vi "Double_GeneralGearShift_WithDeadTime.vi"(6 "error In":errorcluster, 7 "ShifterRef":T1={"DevStatus"={"status"=FALSE, "code"=0, "source"=""}, "Pneumatics Control Module"=0, "Forward Solenoid Channel"=enum."Invalid", "Reverse Solenoid Channel"=enum."Invalid"}, 9 "Shift Value":T3, 10 "Right":dbl, 11 "Left":dbl) -> (0 "error out":errorcluster, 1 "Shifting":bool, 2 "Right Output":dbl, 3 "Left Output":dbl)   [LabVIEW 2017]
uses:
  <vilib>/Rock Robotics/WPI/Solenoid/WPI_SolenoidValue.ctl
  <vilib>/Rock Robotics/WPI/Solenoid/WPI_SolenoidDevRef.ctl
  <vilib>/Rock Robotics/WPI/Solenoid/WPI_SolenoidChannel.ctl
  <vilib>/Rock Robotics/WPI/ThirdParty/Phoenix-LabVIEW/Motor Controller/Controls/CTRE_Phoenix_MotorControl_NeutralMode.ctl
  <vilib>/Rock Robotics/WPI/Solenoid/WPI_SolenoidSetEnum.vi
panel:
  out "Right Starting Point":dbl
  out "Left Starting Point":dbl
  out "TempTimeVal":u32
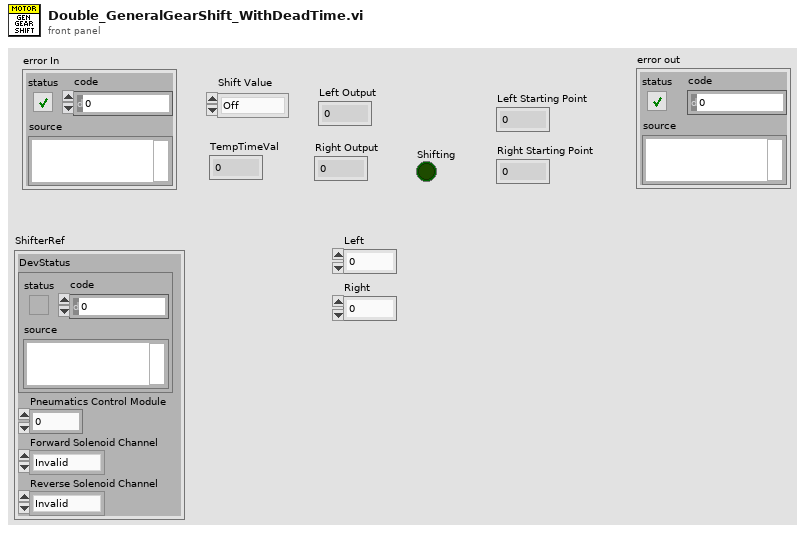
[diagram p1: front panel]
types:
  T1 = typedef "WPI_SolenoidDevRef.ctl" = cluster{"DevStatus":errorcluster, "Pneumatics Control Module":u8, "Forward Solenoid Channel":T2, "Reverse Solenoid Channel":T2}
  T2 = typedef "WPI_SolenoidChannel.ctl" = enum8{"Solenoid 0", "Solenoid 1", "Solenoid 2", "Solenoid 3", "Solenoid 4", "Solenoid 5", "Solenoid 6", "Solenoid 7", "Invalid"}
  T3 = typedef "WPI_SolenoidValue.ctl" = enum16{"Off", "On", "Forward", "Reverse"}
  T4 = typedef "WPI_MotorControlDeviceRef.ctl" = cluster{"DeviceStatus":errorcluster, "Type":T5, "PWM":cluster{"PWM Channel":T6, "DeadBand":T7}, "CAN":cluster{"Device Number":u8, "SetOutput VI Ref":variant, "GetOutput VI Ref":variant, "Enable VI Ref":variant, "Disable VI Ref":variant, "Data":variant}, "Invert":bool, "DIO PWM":cluster{"PWM \"Enable\" Channel":T6, "DIOChannel":T8, "PWM Rate":dbl}}
  T5 = typedef "WPI_MotorControlType.ctl" = enum16{"PWM", "CAN", "DIO PWM"}
  T6 = typedef "FPGA_DIOPWMChannel.ctl" = enum8{"PWM 0", "PWM 1", "PWM 2", "PWM 3", "PWM 4", "PWM 5", "PWM 6", "PWM 7", "PWM 8", "PWM 9", "PWM MXP 0", "PWM MXP 1", "PWM MXP 2", "PWM MXP 3", "PWM MXP 4", "PWM MXP 5", "PWM MXP 6", "PWM MXP 7", "PWM MXP 8", "PWM MXP 9", "Invalid"}
  T7 = typedef "WPI_PWMDeadband.ctl" = cluster{"Name":string, "maxPositivePwm":i32, "minPositivePwm":i32, "centerPwm":i32, "maxNegativePwm":i32, "minNegativePwm":i32, "angularRange":u16}
  T8 = typedef "FPGA_DIOChannel.ctl" = enum8{"DIO 0", "DIO 1", "DIO 2", "DIO 3", "DIO 4", "DIO 5", "DIO 6", "DIO 7", "DIO 8", "DIO 9", "DIO MXP 0", "DIO MXP 1", "DIO MXP 2", "DIO MXP 3", "DIO MXP 4", "DIO MXP 5", "DIO MXP 6", "DIO MXP 7", "DIO MXP 8", "DIO MXP 9", "DIO MXP 10", "DIO MXP 11", "DIO MXP 12", "DIO MXP 13", "DIO MXP 14", "DIO MXP 15", "SPI Port CS1", "SPI Port CS2", "SPI Port CS3", "SPI Port MISO", "SPI Port MOSI", "Invalid"}
  T9 = typedef "CTRE_Phoenix_MotorControl_NeutralMode.ctl" = enum8{"EEPROMSetting", "Override to Coast", "Override to Brake"}
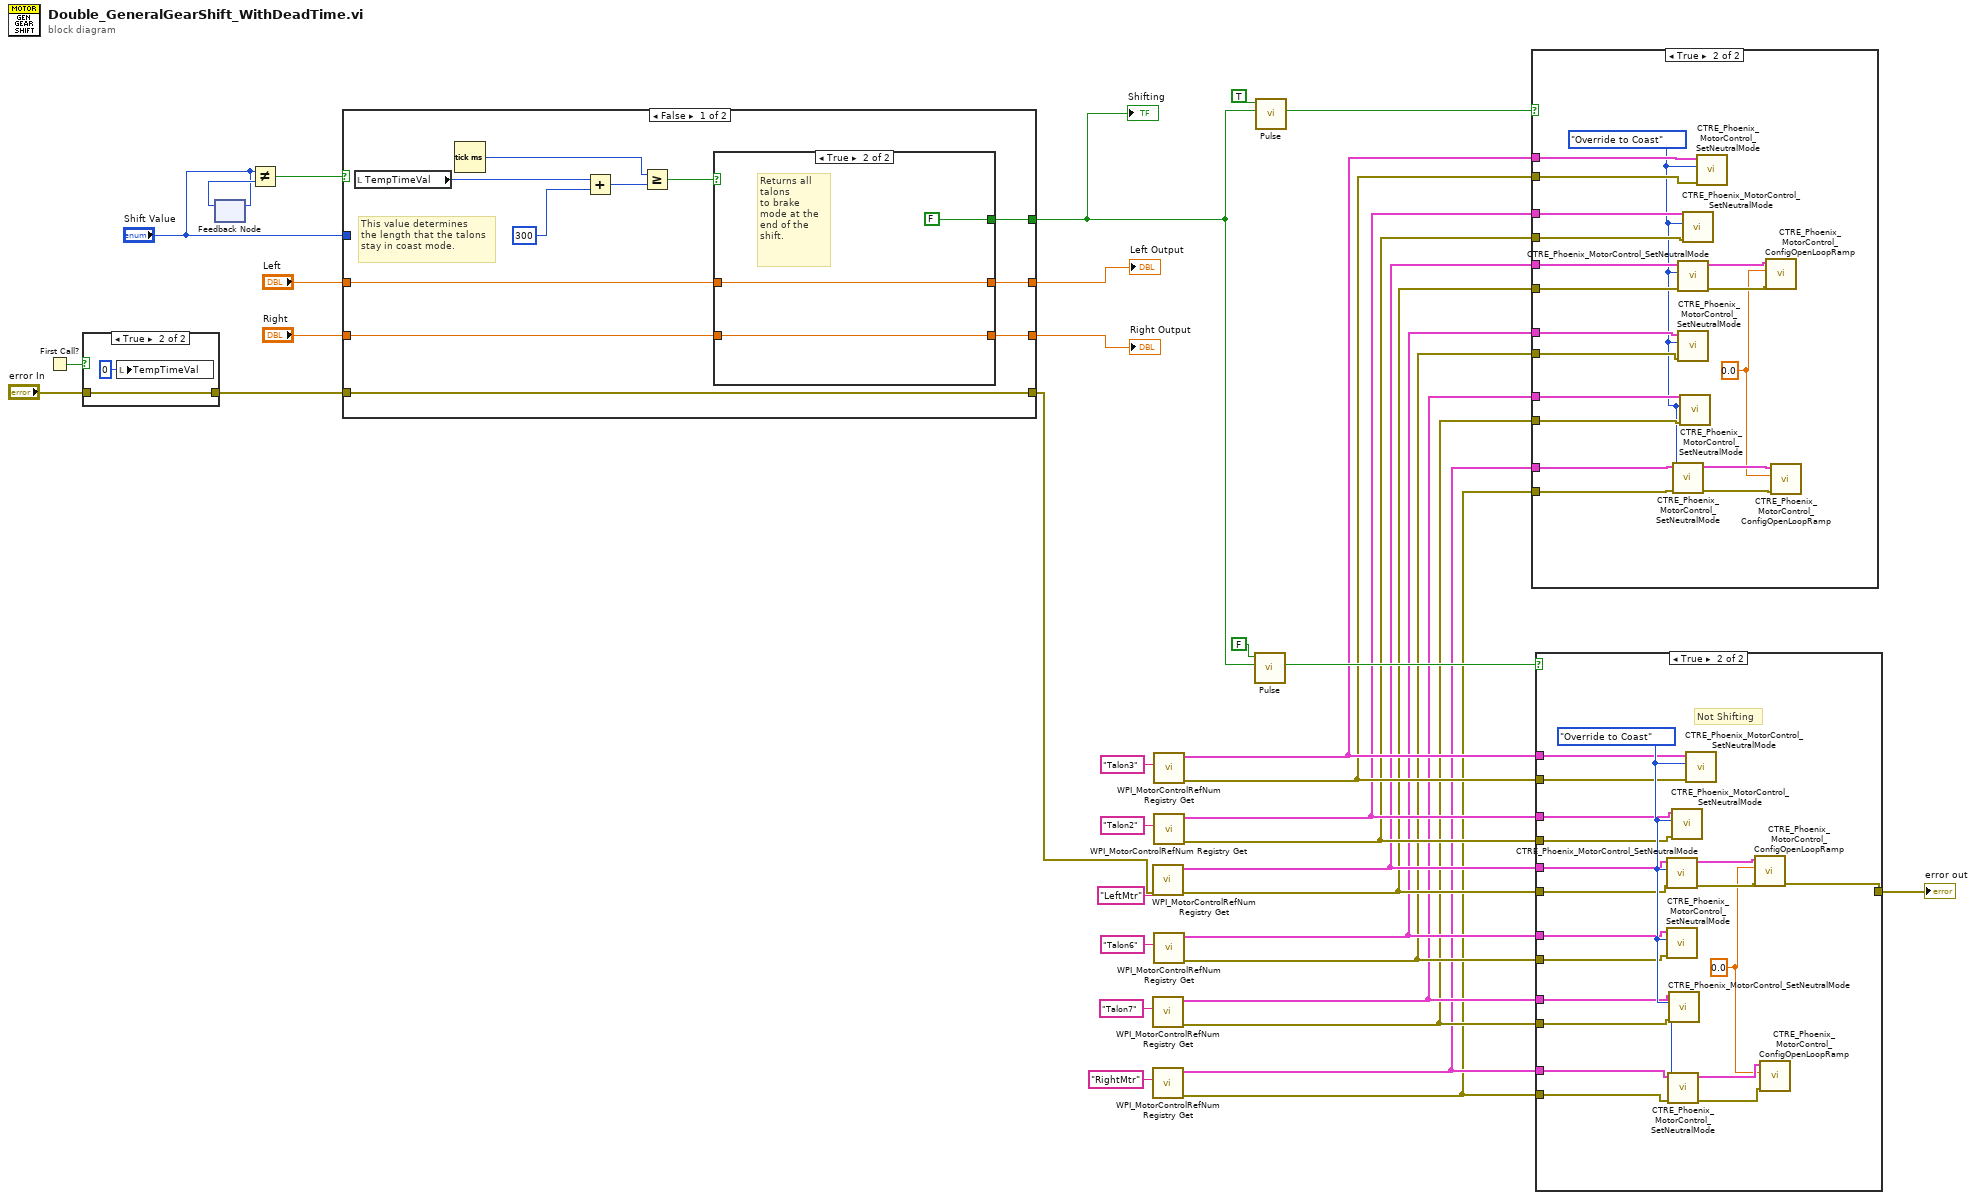
[diagram p0: block diagram]
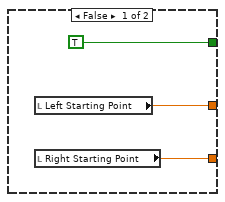
[diagram p5: hidden frame]
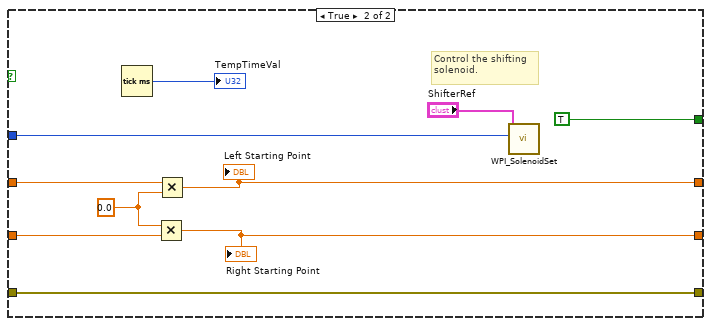
[diagram p6: hidden frame]
diagram:
  n1 = First Call?() -> (First Call?: T/F=w31:bool)
  n2 = case shown="True" w31 {
    tunnel: [w36 w37] -> w3
    tunnel: "error In" -> [w36 w37]
    frame False {
    }
    frame True {
      n3 = local write "TempTimeVal"(u32 0 ("TempTimeVal")) -> ()
    }
  }
  n4 = feedback-in #1("Shift Value") -> ()
  n5 = feedback #1() -> (w29:T3)  [unwired: 1 in]
  n6 = Not Equal?(x="Shift Value", y=w29) -> (x != y?=w28:bool)
  n7 = case shown="False" w28 {
    tunnel: [w49 w61] -> w35
    tunnel: [w48 w60] -> w34
    tunnel: "Right" -> [w47 w63]
    tunnel: "Left" -> [w46 w64]
    tunnel: [w40 TRUE] -> w23
    tunnel: "Shift Value" -> [_ w57]
    tunnel: w3 -> [w39 w56]
    tunnel: [w39 w56] -> w1
    frame False {
      # "This value determines\nthe length that the talons\nstay in coast mode."
      n8 = local read "TempTimeVal"() -> (w42:u32)
      n9 = Tick Count (ms)() -> (millisecond timer value=w44:u32)
      n10 = Add(x=w42, y=300) -> (x+y=w43:u32)
      n11 = Greater Or Equal?(x=w44, y=w43) -> (x >= y?=w45:bool)
      n12 = case shown="True" w45 {
        tunnel: [w51 w54] -> w49
        tunnel: [w52 w55] -> w48
        tunnel: w47 -> [_ w55]
        tunnel: w46 -> [_ w54]
        tunnel: [TRUE FALSE] -> w40
        frame False {
          n13 = local read "Left Starting Point"() -> (w51:dbl)
          n14 = local read "Right Starting Point"() -> (w52:dbl)
        }
        frame True {
          # "Returns all talons\nto brake mode at the\nend of the shift."
        }
      }
    }
    frame True {
      w62 = 0.0
      # "Control the shifting\nsolenoid."
      n15 = Tick Count (ms)() -> (millisecond timer value=→"TempTimeVal":u32)
      n16 = Multiply(x=w62, y=w63) -> (x*y=w60:dbl)
      "Right Starting Point" <- w60
      n17 = Multiply(x=w64, y=w62) -> (x*y=w61:dbl)
      "Left Starting Point" <- w61
      n18 = call-poly <vilib>:"WPI_SolenoidSet.vi"("Value"=w57, "SolenoidDevRef"="ShifterRef") -> ()  [unwired: 8 in, 2 out]
    }
  }
  "Left Output" <- w35
  "Right Output" <- w34
  "Shifting" <- w23
  n19 = call <vilib>:"WPI_MotorControlRefNum Registry Get.vi"("error in (no error)"=w1, "refnum name"="LeftMtr") -> ("error out"=w11:errorcluster, "MotorControlDevRef"=w12:T4)  [unwired: 8 in]
  n20 = call <vilib>:"WPI_MotorControlRefNum Registry Get.vi"("refnum name"="Talon7") -> ("error out"=w7:errorcluster, "MotorControlDevRef"=w8:T4)  [unwired: 9 in]
  n21 = call <vilib>:"WPI_MotorControlRefNum Registry Get.vi"("refnum name"="RightMtr") -> ("error out"=w5:errorcluster, "MotorControlDevRef"=w6:T4)  [unwired: 9 in]
  n22 = call <vilib>:"WPI_MotorControlRefNum Registry Get.vi"("refnum name"="Talon3") -> ("error out"=w15:errorcluster, "MotorControlDevRef"=w16:T4)  [unwired: 9 in]
  n23 = call <vilib>:"WPI_MotorControlRefNum Registry Get.vi"("refnum name"="Talon2") -> ("error out"=w13:errorcluster, "MotorControlDevRef"=w14:T4)  [unwired: 9 in]
  n24 = call <vilib>:"WPI_MotorControlRefNum Registry Get.vi"("refnum name"="Talon6") -> ("error out"=w9:errorcluster, "MotorControlDevRef"=w10:T4)  [unwired: 9 in]
  n25 = call "Pulse.vi"("Input"=w23, "Rising Edge?"=FALSE) -> ("Output"=w25:bool)  [unwired: 9 in]
  n26 = call "Pulse.vi"("Input"=w23, "Rising Edge?"=TRUE) -> ("Output"=w4:bool)  [unwired: 9 in]
  n27 = case shown="True" w4 {
    tunnel: w16 -> [_ w83]
    tunnel: w15 -> [_ w82]
    tunnel: w14 -> [_ w81]
    tunnel: w13 -> [_ w80]
    tunnel: w11 -> [_ w78]
    tunnel: w12 -> [_ w79]
    tunnel: w10 -> [_ w77]
    tunnel: w9 -> [_ w76]
    tunnel: w8 -> [_ w75]
    tunnel: w7 -> [_ w74]
    tunnel: w6 -> [_ w73]
    tunnel: w5 -> [_ w72]
    frame False {
    }
    frame True {
      w71 = CTRE_Phoenix_MotorControl_NeutralMode."Override to Coast" ("Motor Control Neutral Mode")
      w66 = 0.0 ("Throttle Ramp Rate (percent/s)")
      n28 = call <vilib>:"CTRE_Phoenix_MotorControl_SetNeutralMode.vi"("error in (no error)"=w72, "Motor Control Neutral Mode"=w71, "PhoenixMotorControlDevRef"=w73) -> ("error out"=w70:errorcluster, "PhoenixMotorControlDevRef"=w69:T4)  [unwired: 7 in]
      n29 = call <vilib>:"CTRE_Phoenix_MotorControl_SetNeutralMode.vi"("error in (no error)"=w78, "Motor Control Neutral Mode"=w71, "PhoenixMotorControlDevRef"=w79) -> ("error out"=w67:errorcluster, "PhoenixMotorControlDevRef"=w68:T4)  [unwired: 7 in]
      n30 = call <vilib>:"CTRE_Phoenix_MotorControl_SetNeutralMode.vi"("error in (no error)"=w76, "Motor Control Neutral Mode"=w71, "PhoenixMotorControlDevRef"=w77) -> ()  [unwired: 7 in, 2 out]
      n31 = call <vilib>:"CTRE_Phoenix_MotorControl_SetNeutralMode.vi"("error in (no error)"=w74, "Motor Control Neutral Mode"=w71, "PhoenixMotorControlDevRef"=w75) -> ()  [unwired: 7 in, 2 out]
      n32 = call <vilib>:"CTRE_Phoenix_MotorControl_SetNeutralMode.vi"("error in (no error)"=w80, "Motor Control Neutral Mode"=w71, "PhoenixMotorControlDevRef"=w81) -> ()  [unwired: 7 in, 2 out]
      n33 = call <vilib>:"CTRE_Phoenix_MotorControl_SetNeutralMode.vi"("error in (no error)"=w82, "Motor Control Neutral Mode"=w71, "PhoenixMotorControlDevRef"=w83) -> ()  [unwired: 7 in, 2 out]
      n34 = call <vilib>:"CTRE_Phoenix_MotorControl_ConfigOpenLoopRamp.vi"("error in (no error)"=w67, "secondsFromNeutralToFull"=w66, "PhoenixMotorControlDevRef"=w68) -> ()  [unwired: 7 in, 2 out]
      n35 = call <vilib>:"CTRE_Phoenix_MotorControl_ConfigOpenLoopRamp.vi"("error in (no error)"=w70, "secondsFromNeutralToFull"=w66, "PhoenixMotorControlDevRef"=w69) -> ()  [unwired: 7 in, 2 out]
    }
  }
  n36 = case shown="True" w25 {
    tunnel: w16 -> [_ w97]
    tunnel: w15 -> [_ w96]
    tunnel: w14 -> [_ w95]
    tunnel: w13 -> [_ w94]
    tunnel: w11 -> [w84 w92]
    tunnel: w12 -> [_ w93]
    tunnel: w10 -> [_ w91]
    tunnel: w9 -> [_ w90]
    tunnel: w8 -> [_ w89]
    tunnel: w7 -> [_ w88]
    tunnel: w6 -> [_ w87]
    tunnel: w5 -> [_ w86]
    tunnel: [w84 w85] -> w2
    frame False {
    }
    frame True {
      w103 = CTRE_Phoenix_MotorControl_NeutralMode."Override to Coast" ("Motor Control Neutral Mode")
      w98 = 0.0 ("Throttle Ramp Rate (percent/s)")
      # "Not Shifting"
      n37 = call <vilib>:"CTRE_Phoenix_MotorControl_SetNeutralMode.vi"("error in (no error)"=w92, "Motor Control Neutral Mode"=w103, "PhoenixMotorControlDevRef"=w93) -> ("error out"=w99:errorcluster, "PhoenixMotorControlDevRef"=w100:T4)  [unwired: 7 in]
      n38 = call <vilib>:"CTRE_Phoenix_MotorControl_SetNeutralMode.vi"("error in (no error)"=w90, "Motor Control Neutral Mode"=w103, "PhoenixMotorControlDevRef"=w91) -> ()  [unwired: 7 in, 2 out]
      n39 = call <vilib>:"CTRE_Phoenix_MotorControl_SetNeutralMode.vi"("error in (no error)"=w86, "Motor Control Neutral Mode"=w103, "PhoenixMotorControlDevRef"=w87) -> ("error out"=w102:errorcluster, "PhoenixMotorControlDevRef"=w101:T4)  [unwired: 7 in]
      n40 = call <vilib>:"CTRE_Phoenix_MotorControl_SetNeutralMode.vi"("error in (no error)"=w88, "Motor Control Neutral Mode"=w103, "PhoenixMotorControlDevRef"=w89) -> ()  [unwired: 7 in, 2 out]
      n41 = call <vilib>:"CTRE_Phoenix_MotorControl_SetNeutralMode.vi"("error in (no error)"=w94, "Motor Control Neutral Mode"=w103, "PhoenixMotorControlDevRef"=w95) -> ()  [unwired: 7 in, 2 out]
      n42 = call <vilib>:"CTRE_Phoenix_MotorControl_SetNeutralMode.vi"("error in (no error)"=w96, "Motor Control Neutral Mode"=w103, "PhoenixMotorControlDevRef"=w97) -> ()  [unwired: 7 in, 2 out]
      n43 = call <vilib>:"CTRE_Phoenix_MotorControl_ConfigOpenLoopRamp.vi"("error in (no error)"=w99, "secondsFromNeutralToFull"=w98, "PhoenixMotorControlDevRef"=w100) -> ("error out"=w85:errorcluster)  [unwired: 7 in, 1 out]
      n44 = call <vilib>:"CTRE_Phoenix_MotorControl_ConfigOpenLoopRamp.vi"("error in (no error)"=w102, "secondsFromNeutralToFull"=w98, "PhoenixMotorControlDevRef"=w101) -> ()  [unwired: 7 in, 2 out]
    }
  }
  "error out" <- w2
